vi "c_ctre_phoenix6_SetUpdateFrequency.vi"(0 "Numeric 2":i32, 1 "String 2":string, 2 "Numeric 3":u32, 3 "Numeric 4":u16, 4 "Numeric 5":dbl, 5 "Numeric 6":dbl) -> (20 "Numeric":i32, 21 "String":string)   [LabVIEW 2023]
uses:
  <vilib>/Rock Robotics/WPI/ThirdParty/Phoenix-LabVIEW/Controls/DriverLib.ctl
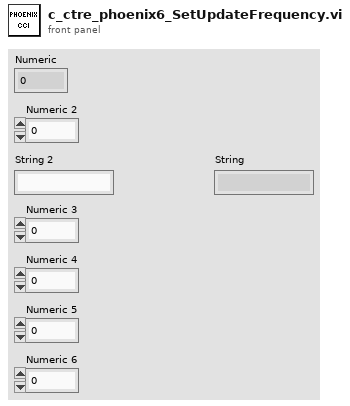
[diagram p1: front panel]
types:
  T1 = typedef "DriverLib.ctl" = path
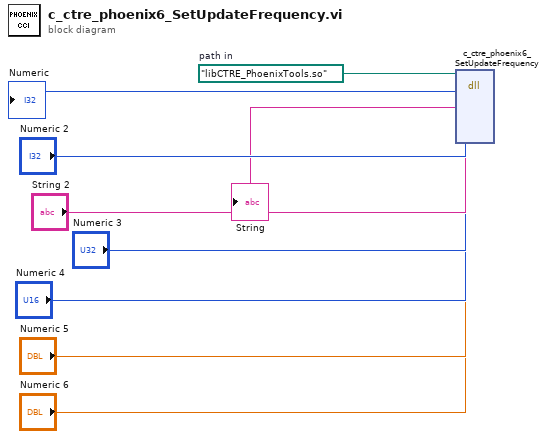
[diagram p0: block diagram]
diagram:
  w9 = T1 path "libCTRE_PhoenixTools.so"  # path in
  n1 = dll-call lib="?" fn="c_ctre_phoenix6_SetUpdateFrequency"(path in=w9, "Numeric 2", "String 2", "Numeric 3", "Numeric 4", "Numeric 5", "Numeric 6") -> (→"Numeric":i32, →"String":string)  [unwired: 7 in, 2 out]
